vi "test Create Message Multiple Devices.vi"(8 "error in (no error)":errorcluster, 11 "TestCase in":refnum<class "Routing and Faulting Unit Tests.lvclass">) -> (0 "error out":errorcluster, 3 "TestCase out":refnum<class "Routing and Faulting Unit Tests.lvclass">)   [LabVIEW 2017, in "Routing and Faulting Unit Tests.lvclass"]
uses:
  Routing and Faulting Unit Tests.lvclass
  Engine/Engine Data.ctl
  Shared/Compiled.Settings.ctl
  Shared/Communication Configuration.ctl
  Shared/Routing and Faulting Configuration.ctl
  Shared/Routing Channel Configuration.ctl
  Shared/Value-Connections Map.ctl
  Shared/Connection.ctl
  Shared/Alias Mapping.ctl
  Shared/FIFO Indices.ctl
  Includes/CDMessaging.lvlibp/Producer/Abstract Producer/Abstract Producer.lvclass
  Engine/Device Inputs.ctl
  Engine/Device Outputs.ctl
  Includes/CDMessaging.lvlibp/Switch/Switch Connect Message/Switch Connect Message.lvclass
  C:/Users/nitest/Documents/ni-official/niveristand-routing-and-faulting-custom-device/Includes/CDMessaging.lvlibp/Message/Abstract Message/Abstract Message.lvclass
  Includes/CDMessaging.lvlibp/Switch/Switch Disconnect Message/Switch Disconnect Message.lvclass
  Engine/Producer Message.ctl
  Includes/CDMessaging.lvlibp/Message/Abstract Message/Abstract Message.lvclass
  <vilib>/addons/_JKI Toolkits/VI Tester/TestCase.llb/TestCase.lvclass
  Engine/Routing and Faulting Engine.lvlib
  Shared/Routing and Faulting Shared.lvlib
  C:/Program Files (x86)/National Instruments/LabVIEW 2017/vi.lib/addons/_JKI Toolkits/VI Tester/TestCase.llb/TestCase.lvclass
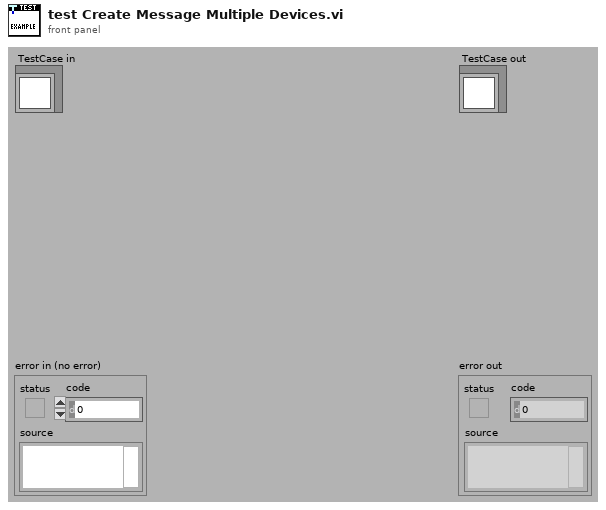
[diagram p1: front panel]
types:
  T1 = typedef "Routing and Faulting Engine.lvlib/Producer Message.ctl" = cluster{"Consumer":string, "Message":refnum<class "Abstract Message.lvclass">}
  T2 = typedef "Routing and Faulting Shared.lvlib/Communication Configuration.ctl" = cluster{"Consumer Queue Names":string[], "Resource Names":string[]}
  T3 = typedef "Routing and Faulting Shared.lvlib/Routing Channel Configuration.ctl" = cluster{"Channel Name":string, "Initial Value":dbl, "FIFO Index":i32, "Value-Connections Map":T4}
  T4 = typedef "Routing and Faulting Shared.lvlib/Value-Connections Map.ctl" = cluster{"State Value Array":i32[], "Connection List Array":cluster{"Connection List":T5[]}[]}
  T5 = typedef "Routing and Faulting Shared.lvlib/Connection.ctl" = cluster{"Resource":string, "Source":string, "Destination":string}
  T6 = typedef "Routing and Faulting Shared.lvlib/Routing and Faulting Configuration.ctl" = cluster{"Routing Channel Configurations":T3[], "Alias Mappings":T7[]}
  T7 = typedef "Routing and Faulting Shared.lvlib/Alias Mapping.ctl" = cluster{"Endpoint":string, "Alias":string}
  T8 = typedef "Routing and Faulting Engine.lvlib/Engine Data.ctl" = cluster{"Compiled.Settings":T9, "Producer":refnum<class "Abstract Producer.lvclass">, "Device Inputs":T11, "Device Outputs":T12, "States Changed":bool[]}
  T9 = typedef "Routing and Faulting Shared.lvlib/Compiled.Settings.ctl" = cluster{"Custom Device Name":string, "Communication Configuration":T2, "Routing and Faulting Configuration":T6, "Status Channels FIFO Indices":T10}
  T10 = typedef "Routing and Faulting Shared.lvlib/FIFO Indices.ctl" = cluster{"Status Channel":i32, "Heartbeat Channel":i32}
  T11 = typedef "Routing and Faulting Engine.lvlib/Device Inputs.ctl" = cluster{"Current Inputs":dbl[], "Previous Inputs":dbl[], "Device Inputs FIFO":refnum<k33>}
  T12 = typedef "Routing and Faulting Engine.lvlib/Device Outputs.ctl" = cluster{"Outputs":dbl[], "Device Outputs FIFO":refnum<k33>}
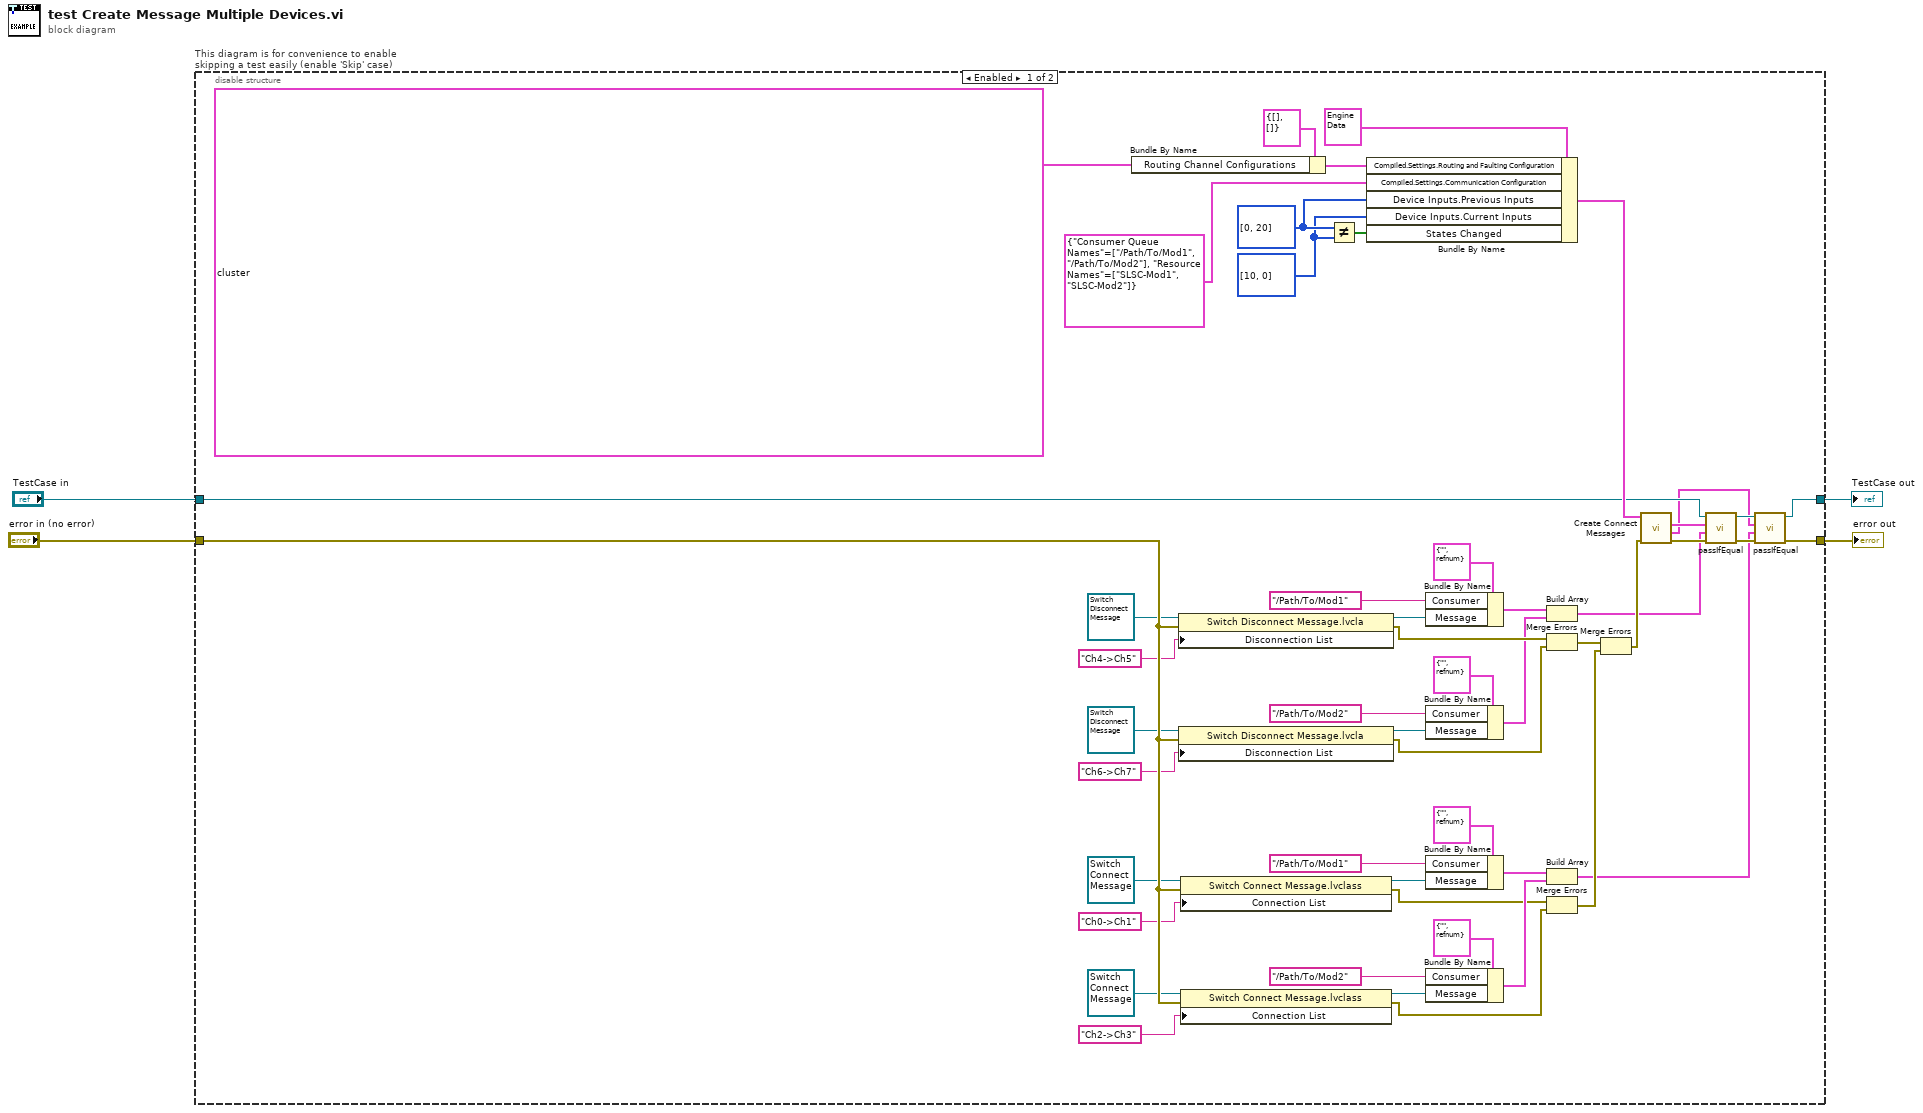
[diagram p0: block diagram]
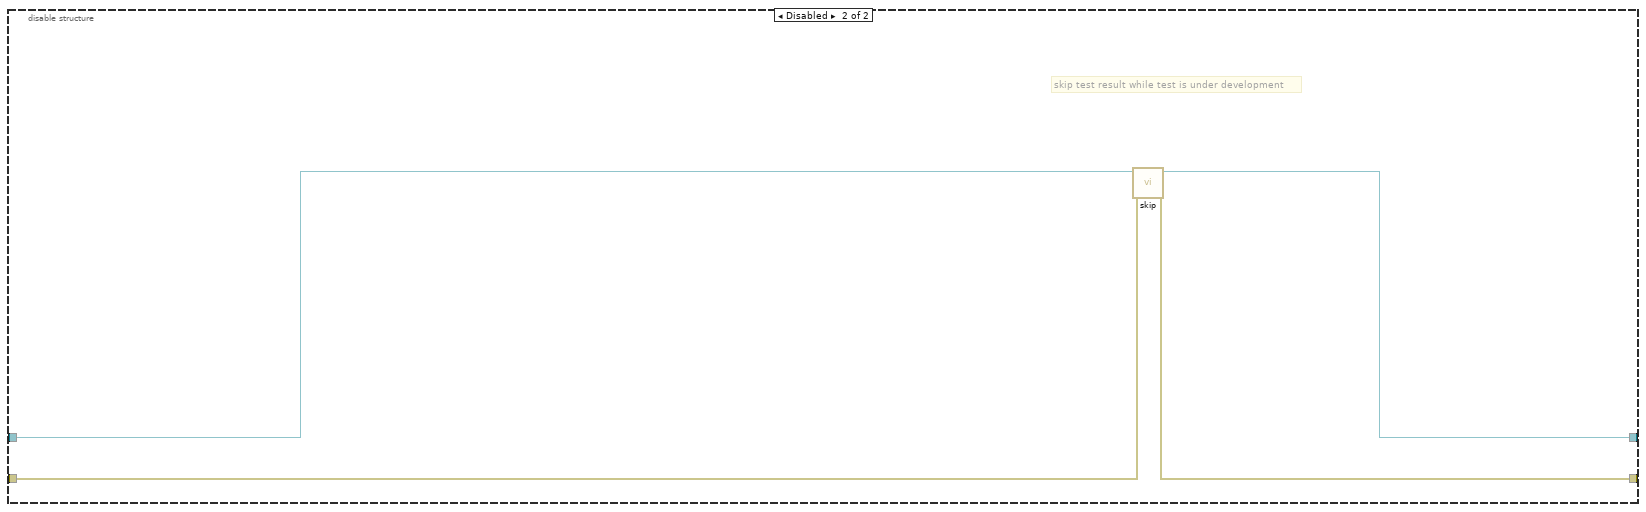
[diagram p2: hidden frame]
diagram:
  n1 = disable-structure "This diagram is for convenience to enable skipping a test easily (enable 'Skip' case)" shown="Enabled" {
    disable-tunnel: "TestCase in" -> [w44 w59]
    disable-tunnel: [w9 w57] -> w1
    disable-tunnel: [w8 w58] -> w3
    disable-tunnel: "error in (no error)" -> [w55 w56]
    frame Enabled {
      w49 = i32[] [10, 0] ("State Value Array")
      w50 = i32[] [0, 20] ("State Value Array")
      n2 = Bundle By Name(cluster=T6 {"Routing Channel Configurations"=[], "Alias Mappings"=[]} ("Compiled.Settings.Routing and Faulting Configuration"), "Routing Channel Configurations"=T3[] [{"Channel Name"="Window Up", "Initial Value"=0.0, "FIFO Index"=0, "Value-Connections Map"={"State Value Array"=[0, 10], "Connection List Array"=[{"Connection List"=[]}, {"Connection List"=[{"Resource"="SLSC-Mod1", "Source"="Ch0", "Destination"="Ch1"}, {"Resource"="SLSC-Mod2", "Source"="Ch2", "Destination"="Ch3"}]}]}}, {"Channel Name"="Window Down", "Initial Value"=0.0, "FIFO Index"=1, "Value-Connections Map"={"State Value Array"=[0, 20], "Connection List Array"=[{"Connection List"=[]}, {"Connection List"=[{"Resource"="SLSC-Mod1", "Source"="Ch4", "Destination"="Ch5"}, {"Resource"="SLSC-Mod2", "Source"="Ch6", "Destination"="Ch7"}]}]}}]) -> (w52:T6)
      n3 = property class="Switch Disconnect Message.lvcla"(reference=refnum<class "Switch Disconnect Message.lvclass"> refnum ("CDMessaging.lvlibp:Switch Disconnect Message.lvclass"), error in=w55, "Disconnection List"="Ch4->Ch5" ("Connection List")) -> (reference out=w17:refnum<class "Switch Disconnect Message.lvclass">, error out=w27:errorcluster)
      n4 = property class="Switch Disconnect Message.lvcla"(reference=refnum<class "Switch Disconnect Message.lvclass"> refnum ("CDMessaging.lvlibp:Switch Disconnect Message.lvclass"), error in=w55, "Disconnection List"="Ch6->Ch7" ("Connection List")) -> (reference out=w23:refnum<class "Switch Disconnect Message.lvclass">, error out=w28:errorcluster)
      n5 = property class="Switch Connect Message.lvclass"(reference=refnum<class "Switch Connect Message.lvclass"> refnum ("CDMessaging.lvlibp:Switch Connect Message.lvclass"), error in=w55, "Connection List"="Ch0->Ch1") -> (reference out=w41:refnum<class "Switch Connect Message.lvclass">, error out=w30:errorcluster)
      n6 = property class="Switch Connect Message.lvclass"(reference=refnum<class "Switch Connect Message.lvclass"> refnum ("CDMessaging.lvlibp:Switch Connect Message.lvclass"), error in=w55, "Connection List"="Ch2->Ch3") -> (reference out=w34:refnum<class "Switch Connect Message.lvclass">, error out=w29:errorcluster)
      n7 = Not Equal?(x=w50, y=w49) -> (x != y?=w48:bool[])
      n8 = Bundle By Name(cluster=T8 {"Compiled.Settings"={"Custom Device Name"="", "Communication Configuration"={"Consumer Queue Names"=[], "Resource Names"=[]}, "Routing and Faulting Configuration"={"Routing Channel Configurations"=[], "Alias Mappings"=[]}, "Status Channels FIFO Indices"={"Status Channel"=0, "Heartbeat Channel"=0}}, "Producer"=refnum, "Device Inputs"={"Current Inputs"=[], "Previous Inputs"=[], "Device Inputs FIFO"=refnum}, "Device Outputs"={"Outputs"=[], "Device Outputs FIFO"=refnum}, "States Changed"=[]} ("Engine Data in"), "Compiled.Settings.Routing and Faulting Configuration"=w52, "Compiled.Settings.Communication Configuration"=T2 {"Consumer Queue Names"=["/Path/To/Mod1", "/Path/To/Mod2"], "Resource Names"=["SLSC-Mod1", "SLSC-Mod2"]}, "Device Inputs.Previous Inputs"=w50, "Device Inputs.Current Inputs"=w49, "States Changed"=w48) -> (w46:T8)
      n9 = Bundle By Name(cluster=T1 {"Consumer"="", "Message"=refnum} ("Producer Message"), "Consumer"="/Path/To/Mod1", "Message"=w17) -> (w19:T1)
      n10 = Bundle By Name(cluster=T1 {"Consumer"="", "Message"=refnum} ("Producer Message"), "Consumer"="/Path/To/Mod2", "Message"=w23) -> (w26:T1)
      n11 = Bundle By Name(cluster=T1 {"Consumer"="", "Message"=refnum} ("Producer Message"), "Consumer"="/Path/To/Mod1", "Message"=w41) -> (w39:T1)
      n12 = Bundle By Name(cluster=T1 {"Consumer"="", "Message"=refnum} ("Producer Message"), "Consumer"="/Path/To/Mod2", "Message"=w34) -> (w31:T1)
      n13 = Build Array(w19, w26) -> (w7:T1[])
      n14 = Merge Errors(w27, w28) -> (w14:errorcluster)
      n15 = Build Array(w39, w31) -> (w5:T1[])
      n16 = Merge Errors(w30, w29) -> (w13:errorcluster)
      n17 = Merge Errors(w14, w13) -> (w12:errorcluster)
      n18 = call "Create Connect Messages.vi"("error in (no error)"=w12, "Engine Data in"=w46) -> ("error out"=w45:errorcluster, "Connect Messages"=w6:T1[], "Disconnect Messages"=w38:T1[])  [unwired: 6 in, 1 out]
      n19 = call-dynamic "passIfEqual.vi"("error in (no error)"=w45, "y"=w7, "x"=w38, "TestCase in"=w44) -> ("error out"=w11:errorcluster, "TestCase out"=w10:refnum<class "Routing and Faulting Unit Tests.lvclass">)  [unwired: 6 in]
      n20 = call-dynamic "passIfEqual.vi"("error in (no error)"=w11, "y"=w5, "x"=w6, "TestCase in"=w10) -> ("error out"=w8:errorcluster, "TestCase out"=w9:refnum<class "Routing and Faulting Unit Tests.lvclass">)  [unwired: 6 in]
    }
    frame Disabled {
      # "skip test result while test is under development"
      n21 = call <vilib>:"skip.vi"("error in (no error)"=w56, "TestCase in"=w59) -> ("error out"=w58:errorcluster, "TestCase out"=w57:refnum<class "Routing and Faulting Unit Tests.lvclass">)  [unwired: 8 in]
    }
  }
  "error out" <- w3
  "TestCase out" <- w1
